vi "niDAQmx Read (Counter DBL 1Chan 1Samp).vi"(0 "task in":refnum<class "Session Factory.lvclass">, 9 "timeout":dbl=10.0 format="%0.2f", 11 "error in":errorcluster) -> (4 "task out":refnum<class "Session Factory.lvclass">, 6 "data":dbl, 15 "error out":errorcluster)   [LabVIEW 2021, in "Session Management niDAQmx.lvlib" / "Session Factory.lvclass"]
doc: "Reads a single floating-point sample from a counter task. Use an instance that reads floating-point values when NI-DAQmx scales counter samples to a floating-point value, such as for frequency and period measurement."
uses:
  Session Factory.lvclass
  Session Factory.lvclass/Session Factory.ctl
  NI DAQmx Client/NI_DAQmx_client.lvlib
  NI DAQmx Client/RPC Messages/nidevice_grpc_Session.ctl
  NI DAQmx Client/RPC Messages/nidaqmx_grpc_ReadCounterScalarF64Request.ctl
  NI DAQmx Client/RPC Messages/nidevice_grpc_Session_session/nidevice_grpc_Session_session.lvclass
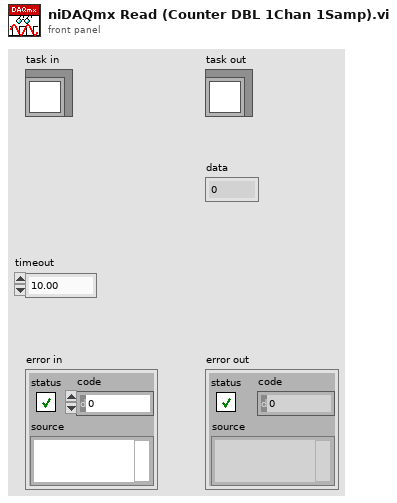
[diagram p1: front panel]
types:
  T1 = typedef "NI_DAQmx_client.lvlib/nidaqmx_grpc_ReadCounterScalarF64Request.ctl" = cluster{"task":T2, "timeout":dbl}
  T2 = typedef "NI_DAQmx_client.lvlib/nidevice_grpc_Session.ctl" = cluster{"nidevice_grpc_Session_session":refnum<class "nidevice_grpc_Session_session.lvclass">}
  T3 = typedef "grpc-lvsupport-release.lvlib/grpcId.ctl" = u64
  T4 = typedef "NI_DAQmx_client.lvlib/nidaqmx_grpc_ReadCounterScalarF64Response.ctl" = cluster{"status":i32, "value":dbl}
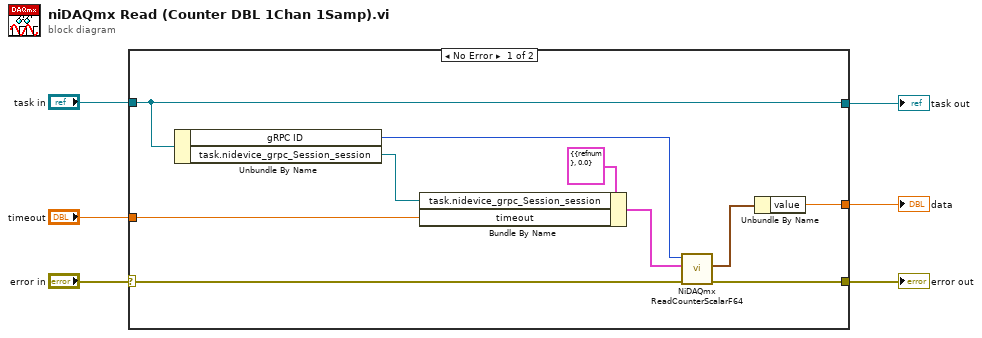
[diagram p0: block diagram]
diagram:
  n1 = case shown="No Error" "error in" {
    selector: "error in" -> [w16 w18]
    tunnel: [w15 w18] -> w5
    tunnel: "task in" -> [w14 w17]
    tunnel: [w14 w17] -> w3
    tunnel: "timeout" -> [w9 _]
    tunnel: [w7 _] -> w1
    frame No Error {
      n2 = Unbundle By Name(w14) -> ("gRPC ID"=w12:T3, "task.nidevice_grpc_Session_session"=w11:refnum<class "nidevice_grpc_Session_session.lvclass">)
      n3 = Bundle By Name(cluster=T1 {"task"={"nidevice_grpc_Session_session"=refnum}, "timeout"=0.0} ("Request Data"), "task.nidevice_grpc_Session_session"=w11, "timeout"=w9) -> (w10:T1)
      n4 = call "NiDAQmx ReadCounterScalarF64.vi"("error in"=w16, "Request Data"=w10, "gRPC ID"=w12) -> ("error out"=w15:errorcluster, "Response Data"=w8:T4)  [unwired: 6 in, 1 out]
      n5 = Unbundle By Name(w8) -> ("value"=w7:dbl)
    }
    frame Error {
    }
  }
  "error out" <- w5
  "task out" <- w3
  "data" <- w1
